vi "Add Database.vi"(7 "Highlight? (F)":bool, 8 "error in":errorcluster, 9 "Path":path, 10 "Name":string, 11 "Database section Ref":T1 format="%.0x") -> (0 "error out":errorcluster, 3 "Database Ref out":T1 format="%.0x")   [LabVIEW 2020, in "Communication Bus Template Scripting.lvlib"]
uses:
  <vilib>/NI VeriStand/Custom Device API/Custom Device Item Ref.ctl
  Constants.vi
  Communication Bus Template Scripting.lvlib
  <vilib>/NI VeriStand/Custom Device API/Custom Device API.lvlib
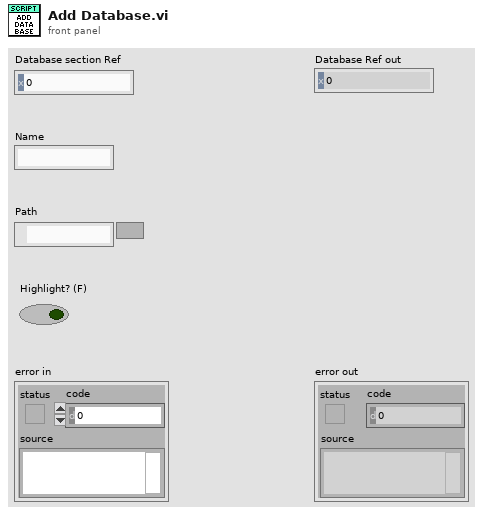
[diagram p1: front panel]
types:
  T1 = typedef "Custom Device API.lvlib/Custom Device Item Ref.ctl" = u64
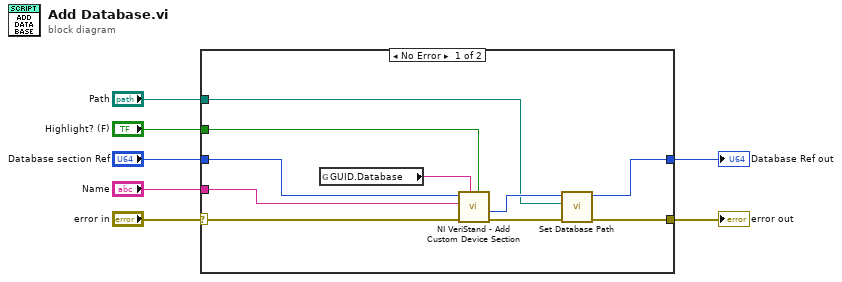
[diagram p0: block diagram]
diagram:
  n1 = case shown="No Error" "error in" {
    selector: "error in" -> [w10 w19]
    tunnel: "Name" -> [w15 _]
    tunnel: "Database section Ref" -> [w14 w18]
    tunnel: [w13 w19] -> w5
    tunnel: "Path" -> [w12 _]
    tunnel: "Highlight? (F)" -> [w11 _]
    tunnel: [w9 w18] -> w1
    frame No Error {
      n2 = global read "Constants.vi" "GUID.Database"() -> (w8:string)
      n3 = call <vilib>:"NI VeriStand - Add Custom Device Section.vi"("Highlight? (F)"=w11, "GUID (Default Section)"=w8, "error in (no error)"=w10, "Section Name"=w15, "Parent Ref in"=w14) -> ("error out"=w16:errorcluster, "Section Ptr"=w17:T1)  [unwired: 3 in, 2 out]
      n4 = call "Set Database Path.vi"("error in"=w16, "Path"=w12, "Database Ref"=w17) -> ("error out"=w13:errorcluster, "Database Ref out"=w9:T1)  [unwired: 7 in]
    }
    frame Error {
    }
  }
  "error out" <- w5
  "Database Ref out" <- w1
